vi "IPS Read PS Current.vi"(4 "Error In":errorcluster, 7 "VISA resource name":refnum<visa-resource-name>="COM3") -> (0 "Error Out":errorcluster, 1 "Current (A)":dbl, 2 "read buffer":string, 3 "VISA resource name":refnum<visa-resource-name>="GPIB1::25::INSTR")   [LabVIEW 2016, in "IPS-120.lvlib"]
uses:
  IPS-120.lvlib
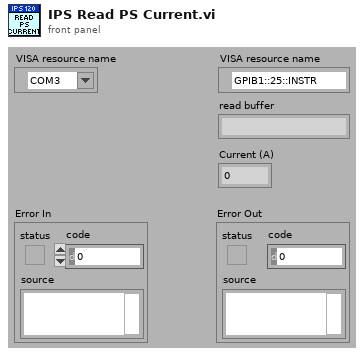
[diagram p1: front panel]
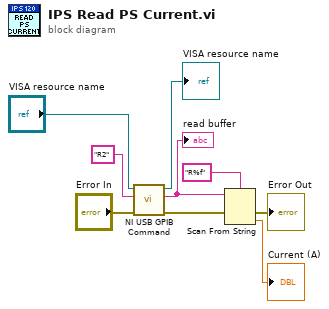
[diagram p0: block diagram]
diagram:
  n1 = call "NI USB GPIB Command.vi"("Error In"="Error In", "write buffer"="R2" ("String to Send"), "VISA resource name"="VISA resource name") -> ("Error Out"=w2:errorcluster, "read buffer"=w5:string, "VISA resource name out"=→"VISA resource name":refnum<visa-resource-name>)  [unwired: 6 in]
  "read buffer" <- w5
  n2 = Scan From String(format string="R%f", input string=w5, error in=w2) -> (error out=→"Error Out":errorcluster, output 1=→"Current (A)":dbl)  [unwired: 1 in, 3 out]
